vi "waitTest.vi"() -> ()   [LabVIEW 2016]
uses:
  <vilib>/FPGAPlugInAG/roboRIO/niLvFpga_Open_roboRIO.vi
  <vilib>/rvi/interface/common/dynamic/niFpgaDynamicAddResources.vi
  <vilib>/FPGAPlugInAG/Dynamic/niLvFpga_Reset_Dynamic.vi
  <vilib>/myRIO/Common/Instrument Driver Framework/Utilities/vis/FPGA Ref Manager.vi
  <vilib>/Utility/error.llb/Error Cluster From Error Code.vi
  <vilib>/myRIO/Common/Instrument Driver Framework/Utilities/vis/Ref Counter.vi
  <vilib>/FPGAPlugInAG/Dynamic/niLvFpga_Run_Dynamic.vi
  GlobalVI.vi
  <vilib>/myRIO/Common/Instrument Driver Framework/roboRIO v1.0/AO/vis/roboRIO v1.0 Write AO.vi
  <vilib>/FPGAPlugInAG/Dynamic/niLvFpga_Close_Dynamic.vi
  <vilib>/rvi/interface/nirviOpenFPGA/nirviOpenFPGA.xnode
  FPGA/FPGA Bitfiles/UnicornMain_FPGATarget_MainFPGAcode_pijQzTnE6Wg.lvbitx
  <vilib>/rvi/interface/nirviMethod/nirviMethod.xnode
  <vilib>/rvi/interface/nirviCloseFPGA/nirviCloseFPGA.xnode
  <vilib>/myRIO/Instrument Drivers/Onboard IO/AO/AO.lvlib
  <vilib>/myRIO/Instrument Drivers/Utilities/Utilities.lvlib
  <vilib>/FPGAPlugInAG/Dynamic/niLvFpga_StartFifo_Dynamic.vi
  <vilib>/rvi/errors/niLvFpgaMergeErrorWithErrorCode.vi
panel:
  out "FPGA REF Error out":errorcluster
  out "error out":errorcluster
  in  "error in (no error)":errorcluster
  in  "B/AO0 (Pin 2)":dbl
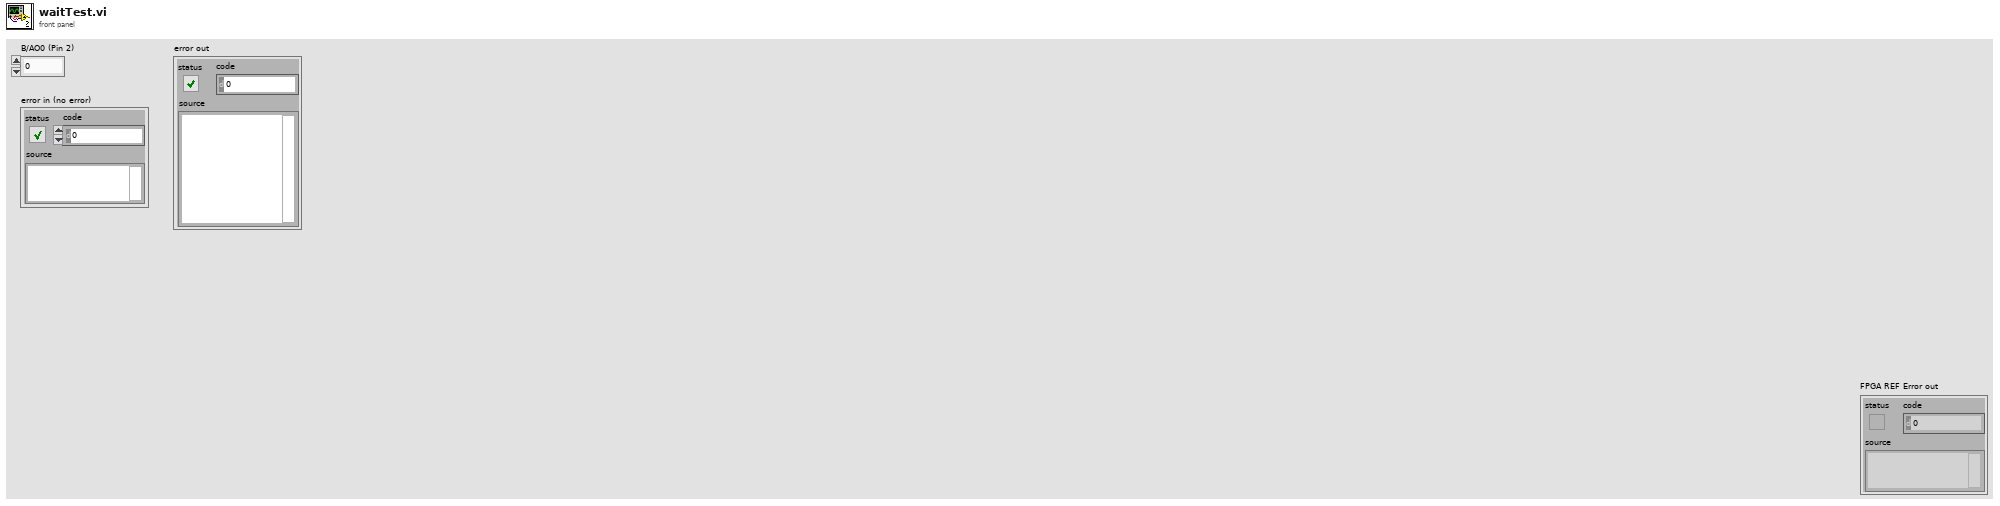
[diagram p1: front panel]
types:
  T1 = typedef "AO.lvlib/AO Reference.ctl" = cluster{"myRIO Reference":T2, "AO Channel List":T6, "AO Scaling Constant List":T8}
  T2 = typedef "myRIO Generic Hardware Reference.ctl" = cluster{"myRIO Model":T3, "myRIO Hardware Reference":T4}
  T3 = typedef "Hardware Version Enum.ctl" = enum16{"Unknown", "myRIO-1900", "myRIO-1950", "roboRIO", "NI ELVIS RIO CM"}
  T4 = typedef "myRIO v1.0 Reference.ctl" = cluster{"Generic FPGA Reference":T5, "Allow multiple opens":bool}
  T5 = typedef "Generic FPGA Reference.ctl" = refnum<k20>
  T6 = typedef "AO Channels List.ctl" = T7[]
  T7 = typedef "AO Channels Enum.ctl" = enum16{"Not Connected", "AudioOut/Left", "AudioOut/Right", "C/AO0", "C/AO1", "A/AO0", "A/AO1", "B/AO0", "B/AO1"}
  T8 = typedef "Analog Scaling Constants List.ctl" = T9[]
  T9 = typedef "Analog Scaling Constants.ctl" = cluster{"LSB Weight (Volts)":dbl, "Offset (Volts)":dbl, "Signed?":bool}
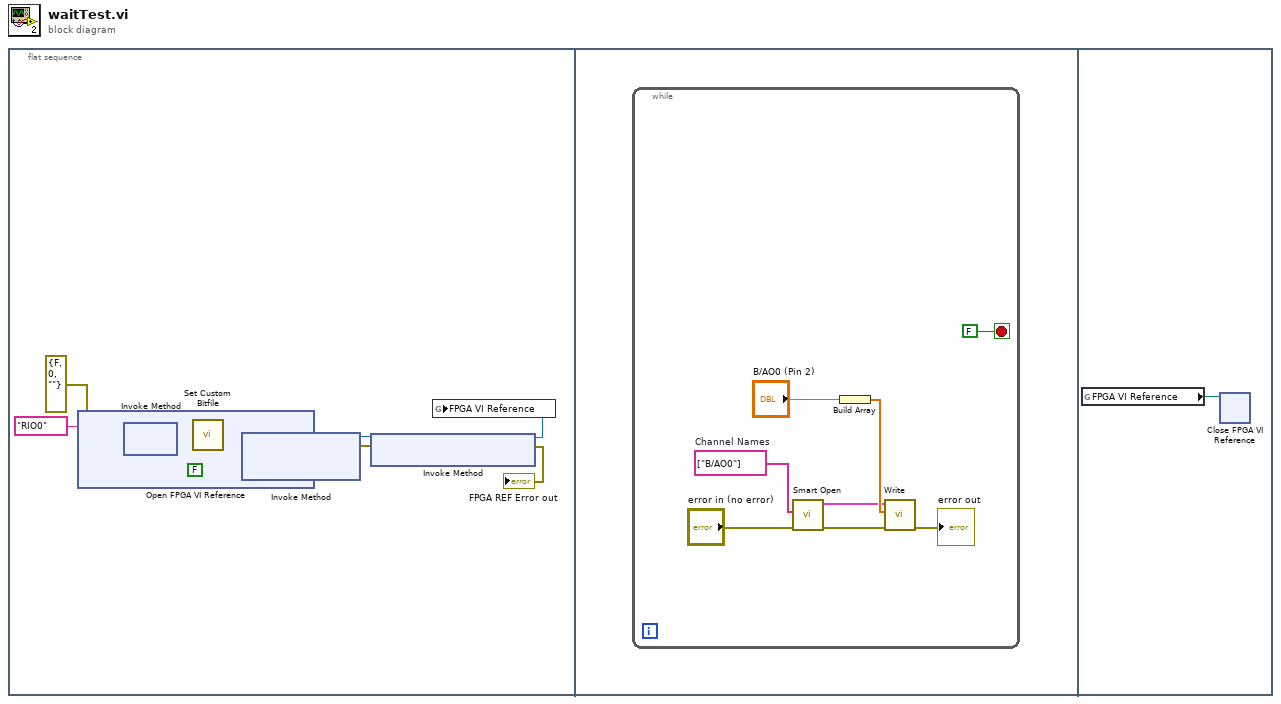
[diagram p0: block diagram]
diagram:
  n1 = flat-sequence {
    frame #0 {
      n2 = xnode "Open FPGA VI Reference"("error in"=errorcluster {"status"=FALSE, "code"=0, "source"=""}, "resource name"=tag "RIO0") -> ("FPGA VI Reference Out"=w8:refnum<k20>, "error out"=w7:errorcluster)
      n3 = xnode "Invoke Method"("FPGA VI Reference In"=w8, "error in"=w7) -> ("FPGA VI Reference Out"=w4:refnum<k20>, "error out"=w5:errorcluster)
      n4 = call <vilib>:"Set Custom Bitfile.vi"("error in (no error)"=w5, "Custom FPGA Reference In"=w4) -> ("error out"=w3:errorcluster, "Custom FPGA Reference Out"=w2:refnum<k20>)  [unwired: 8 in]
      n5 = xnode "Invoke Method"("FPGA VI Reference In"=w2, "error in"=w3, "Wait Until Done (F)"=FALSE) -> ("FPGA VI Reference Out"=w10:refnum<k20>, "error out"=w11:errorcluster)
      n6 = xnode "Invoke Method"("FPGA VI Reference In"=w10, "error in"=w11) -> ("FPGA VI Reference Out"=w12:refnum<k20>, "error out"=→"FPGA REF Error out":errorcluster)
      n7 = global write "GlobalVI.vi" "FPGA VI Reference"(w12) -> ()
    }
    frame #1 {
      n8 = while {
        stop <- FALSE stop-if-true
        w20 = tag[] ["B/AO0"]  # Channel Names
        n9 = call <vilib>:"Smart Open.vi"("error in (no error)"="error in (no error)", "Channel Names"=w20) -> ("error out"=w15:errorcluster, "AO Ref Out"=w16:T1)  [unwired: 8 in]
        n10 = Build Array("B/AO0 (Pin 2)") -> (w19:dbl[])
        n11 = call <vilib>:"Write.vi"("error in (no error)"=w15, "Values"=w19, "AO Ref In"=w16) -> ("error out"=→"error out":errorcluster)  [unwired: 6 in, 1 out]
      }
    }
    frame #2 {
      n12 = global read "GlobalVI.vi" "FPGA VI Reference"() -> (w22:refnum<k20>)
      n13 = xnode "Close FPGA VI Reference"("FPGA VI Reference In"=w22) -> ()  [unwired: 1 in, 1 out]
    }
  }
